vi "HHGetCountRates.vi"(0 "DeviceIndex":i32) -> (1 "SyncRate":i32, 2 "Error":bool, 3 "Rate 1":i32, 4 "Rate 2":i32, 5 "Rate 3":i32, 6 "Rate 4":i32)   [LabVIEW 2009]
uses:
  hhlib.dll
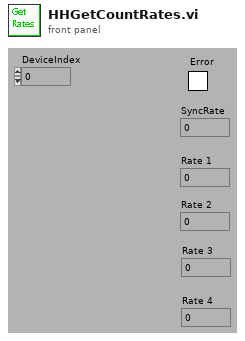
[diagram p1: front panel]
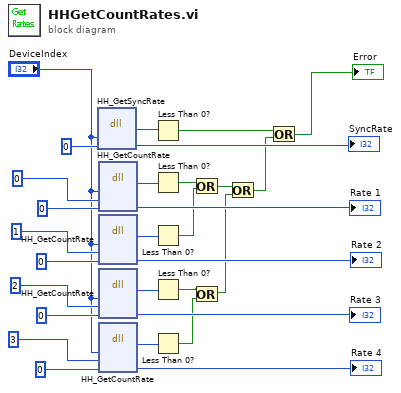
[diagram p0: block diagram]
diagram:
  n1 = dll-call lib="C:/Programme/Anwendungen/DAQLinescan_HH/hhlib.dll" fn="HH_GetSyncRate"("devidx"="DeviceIndex", "rate"=0) -> (w28:i32, "rate"=→"SyncRate":i32)  [unwired: 4 in, 2 out]
  n2 = dll-call lib="C:/Programme/Anwendungen/DAQLinescan_HH/hhlib.dll" fn="HH_GetCountRate"("devidx"="DeviceIndex", "channel"=0, "rate"=0) -> (w21:i32, "rate"=→"Rate 1":i32)  [unwired: 5 in, 2 out]
  n3 = dll-call lib="C:/Programme/Anwendungen/DAQLinescan_HH/hhlib.dll" fn="HH_GetCountRate"("devidx"="DeviceIndex", "channel"=1, "rate"=0) -> (w18:i32, "rate"=→"Rate 2":i32)  [unwired: 5 in, 2 out]
  n4 = dll-call lib="C:/Programme/Anwendungen/DAQLinescan_HH/hhlib.dll" fn="HH_GetCountRate"("devidx"="DeviceIndex", "channel"=2, "rate"=0) -> (w13:i32, "rate"=→"Rate 3":i32)  [unwired: 5 in, 2 out]
  n5 = dll-call lib="C:/Programme/Anwendungen/DAQLinescan_HH/hhlib.dll" fn="HH_GetCountRate"("devidx"="DeviceIndex", "channel"=3, "rate"=0) -> (w10:i32, "rate"=→"Rate 4":i32)  [unwired: 5 in, 2 out]
  n6 = Less Than 0?(x=w28) -> (x < 0?=w27:bool)
  n7 = Less Than 0?(x=w21) -> (x < 0?=w29:bool)
  n8 = Less Than 0?(x=w18) -> (x < 0?=w5:bool)
  n9 = Less Than 0?(x=w13) -> (x < 0?=w7:bool)
  n10 = Less Than 0?(x=w10) -> (x < 0?=w6:bool)
  n11 = Or(x=w29, y=w5) -> (x .or. y?=w4:bool)
  n12 = Or(x=w7, y=w6) -> (x .or. y?=w3:bool)
  n13 = Or(x=w4, y=w3) -> (x .or. y?=w2:bool)
  n14 = Or(x=w27, y=w2) -> (x .or. y?=→"Error":bool)
